vi "Test v2 Client.vi"() -> ()   [LabVIEW 2020]
uses:
  InfluxDB v2 Client/Client/Header-Body Data.ctl
  InfluxDB v2 Client/Client/Error Handler/HTTP Status.ctl
  InfluxDB v2 Client/Client/DataBase Data.ctl
  InfluxDB v2 Client/Data Point/Tag.ctl
  Field Values.ctl
  InfluxDB v2 Client/Client/Write Precision.ctl
  InfluxDB v2 Client/Client/Influx Command.ctl
  Setup/Setup Data.ctl
  InfluxDB v2 Client/Data Point/Data Point - Cmd.ctl
  InfluxDB v2 Client/Client/Write Data.ctl
  <vilib>/Utility/xml.llb/Read From XML File(string).vi
  <vilib>/Utility/xml.llb/Write to XML File(string).vi
  InfluxDB v2 Client/InfluxDB v2 Client.lvlib
panel:
  out "Response":T1
  in  "Tab Control":enum32{"Setup", "Init ", "Write", "Query"}(tab)
  in  "Write Setup":bool
  in  "Read Setup":bool
  in  "File Path Setup":path
  in  "Init":bool
  in  "Check Auth":bool
  in  "DataBase Data":T2
  in  "Timestamp precision":T3=enum."Seconds"
  in  "Measurement":string
  in  "Bucket":string
  in  "Init Data Point":bool
  in  "Write Data":bool
  in  "Field Names":string[](array[string])=["cpu_temp", "error_code", "cpu_load", "cpu_type", "cpu_busy"]
  in  "Tags":T4[](array[typedef])=[{"Key"="host1", "Value"="myPC"}, {"Key"="host2", "Value"="X-Server"}]
  in  "Field Values":T5={"cpu_temp"=48.25, "error_code"=-9003, "cpu_load"=8, "cpu_type"="Ryzen 5 2600", "cpu_busy?"=FALSE}
  in  "Write Query":bool
  in  "Read Query":bool
  in  "with compression?":bool
  in  "Write csv - file":bool
  in  "Query":string="from(bucket: \"Test\")\n  |> range(start: -30m)\n  |> filter(fn: (r) => r[\"_measurement\"] == \"mem3\")\n  |> filter(fn: (r) => r[\"_field\"] == \"cpu_temp\")\n  |> aggregateWindow(every: 1s, fn: last, createEmpty: false)\n  |> yield(name: \"last\")"
  in  "Query Data":bool
  in  "File Path Queries":path
  out "HTTP Status":T6
  in  "Stop":bool
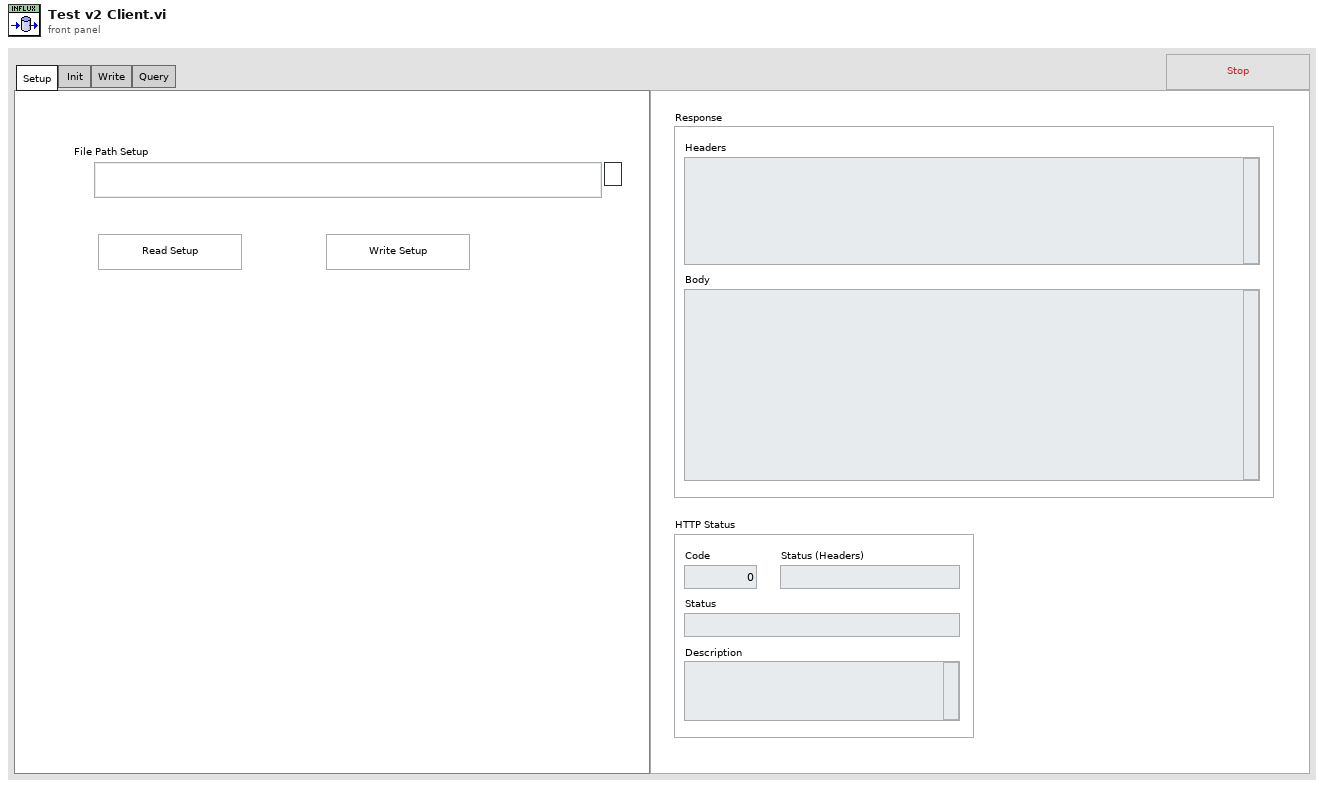
[diagram p1: front panel]
types:
  T1 = typedef "InfluxDB v2 Client.lvlib/Header-Body Data.ctl" = cluster{"Headers":string, "Body":string}
  T2 = typedef "InfluxDB v2 Client.lvlib/DataBase Data.ctl" = cluster{"Api Token":string, "Organization":string, "url":string, "Organization ID":string}
  T3 = typedef "InfluxDB v2 Client.lvlib/Write Precision.ctl" = enum16{"Nanoseconds", "Microseconds", "Milliseconds", "Seconds"}
  T4 = typedef "InfluxDB v2 Client.lvlib/Tag.ctl" = cluster{"Key":string, "Value":string}
  T5 = typedef "Field Values.ctl" = cluster{"cpu_temp":dbl, "error_code":i64, "cpu_load":u64, "cpu_type":string, "cpu_busy?":bool}
  T6 = typedef "InfluxDB v2 Client.lvlib/HTTP Status.ctl" = cluster{"Code":i32, "Status":string, "Description":string, "Status (Headers)":string}
  T7 = typedef "InfluxDB v2 Client.lvlib/Influx Command.ctl" = enum16{"Init", "Check Auth", "Query Data", "Query ZIP Data", "Write Data", "Close"}
  T8 = enum16{"open", "replace", "create", "open or create", "replace or create", "replace or create with confirmation"}
  T9 = typedef "InfluxDB v2 Client.lvlib/Data Point - Cmd.ctl" = enum16{"Init", "Add Tags", "Add Fields", "Add Field Names", "Add Field Values", "Add Measurement", "Add Time Stamp", "Add Precision", "Get Line Protocol"}
  T10 = typedef "Setup Data.ctl" = cluster{"DataBase Data":T2, "Query - csv":string, "Bucket":string, "Measurement":string, "Timestamp precision":T3, "Tags":T4[]}
  T11 = typedef "InfluxDB v2 Client.lvlib/Write Data.ctl" = cluster{"Bucket":string, "Timestamp precision":T3, "Line protocol":string}
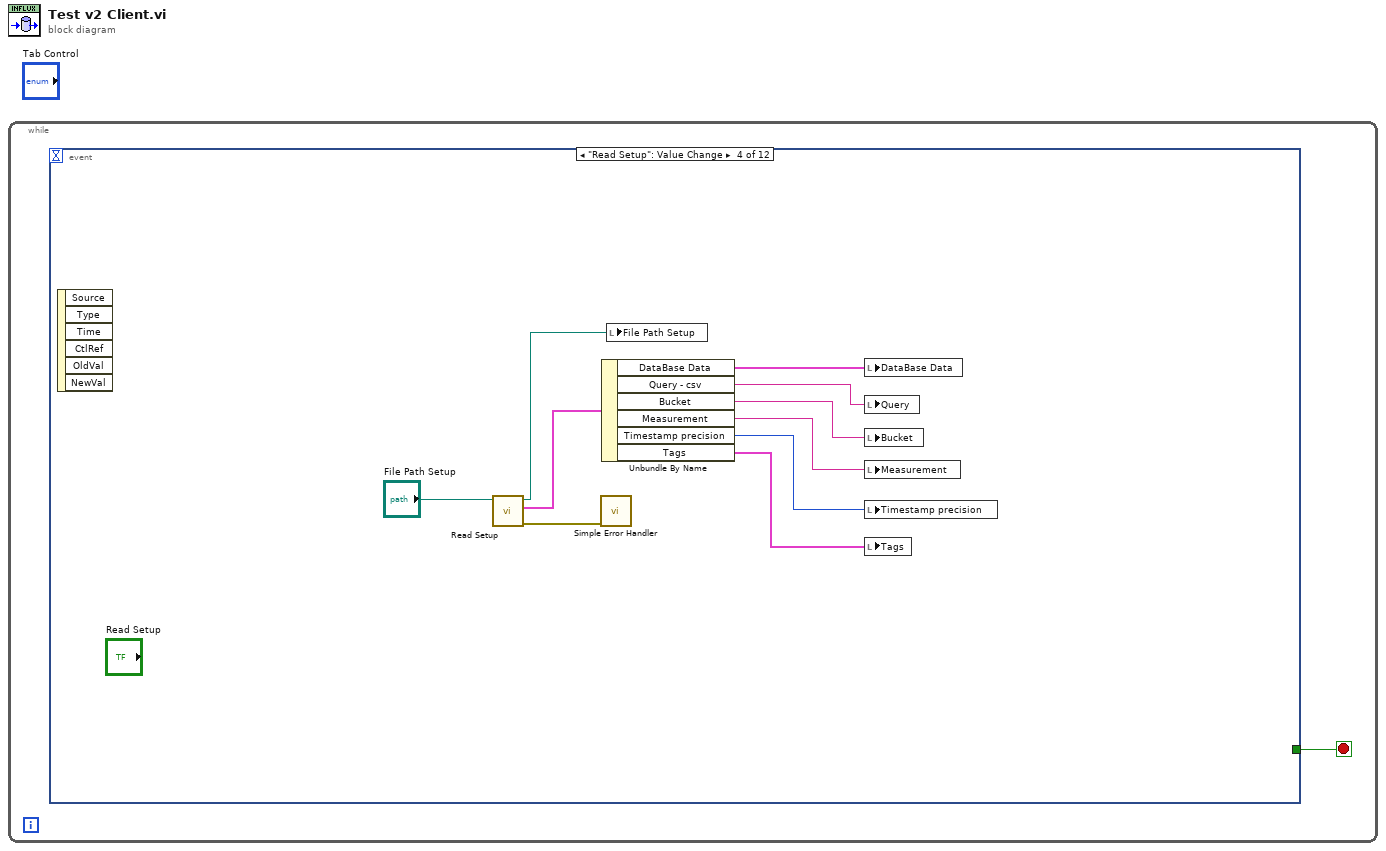
[diagram p0: block diagram]
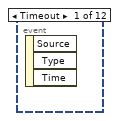
[diagram p2: hidden frame]
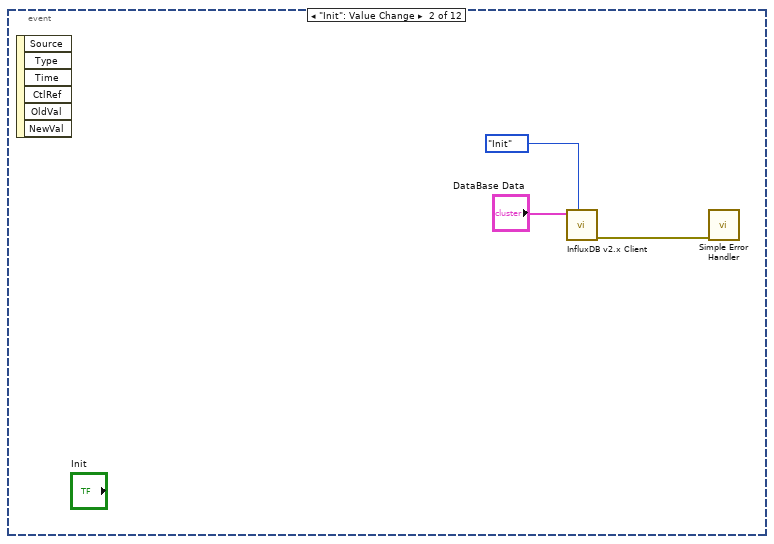
[diagram p3: hidden frame]
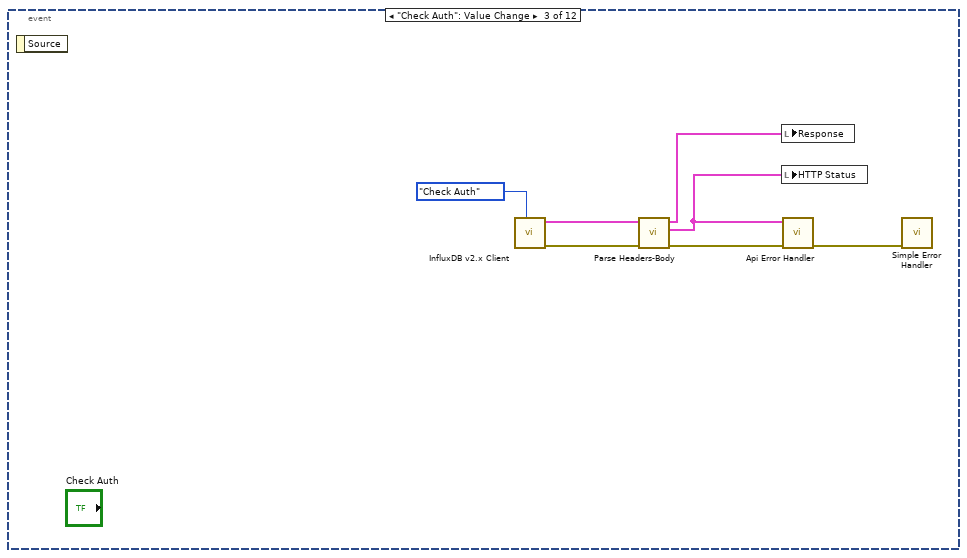
[diagram p4: hidden frame]
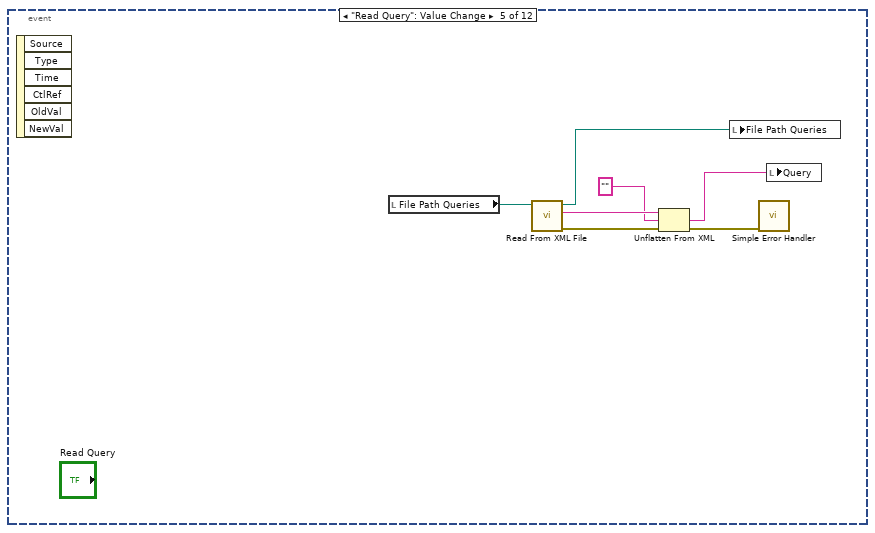
[diagram p5: hidden frame]
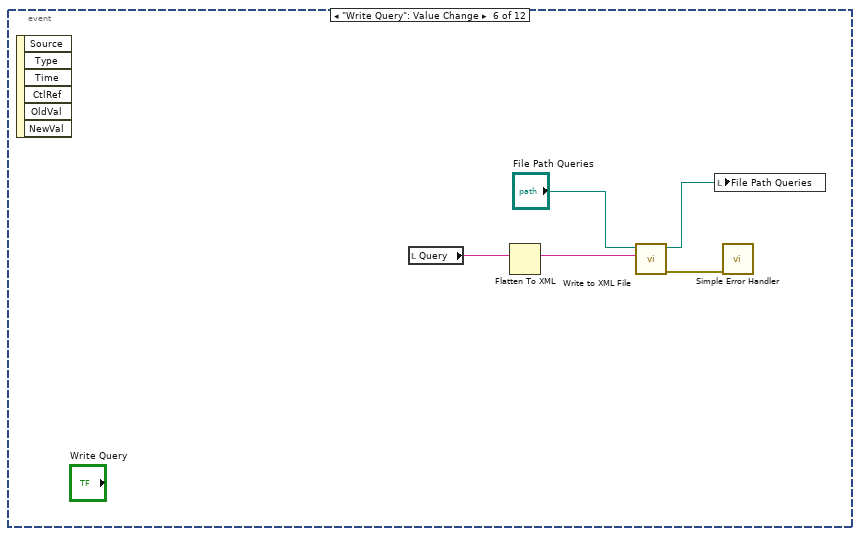
[diagram p6: hidden frame]
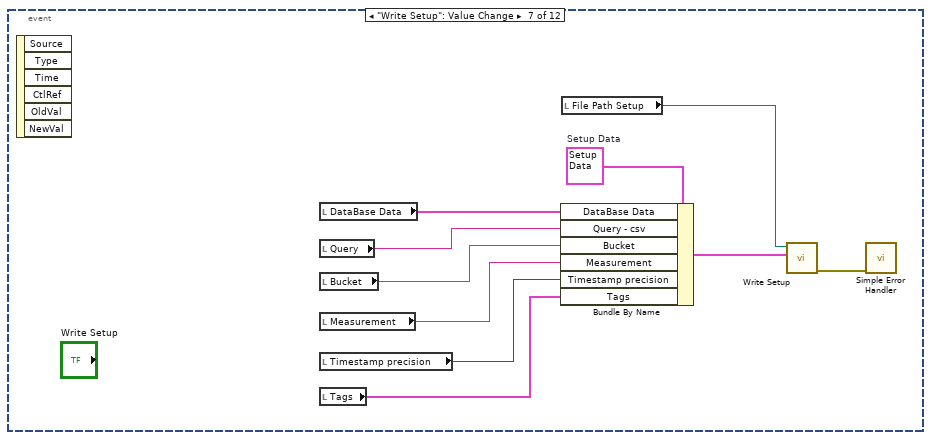
[diagram p7: hidden frame]
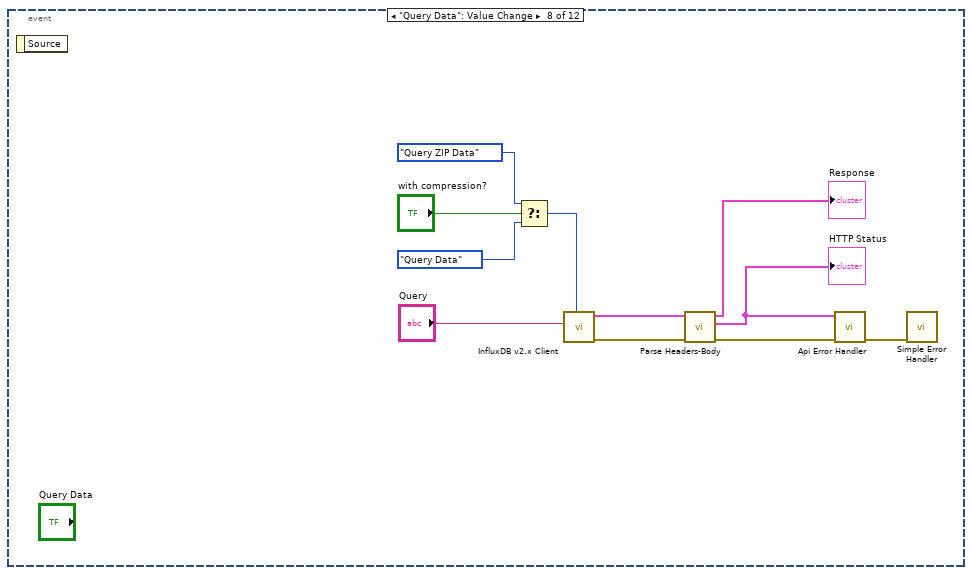
[diagram p8: hidden frame]
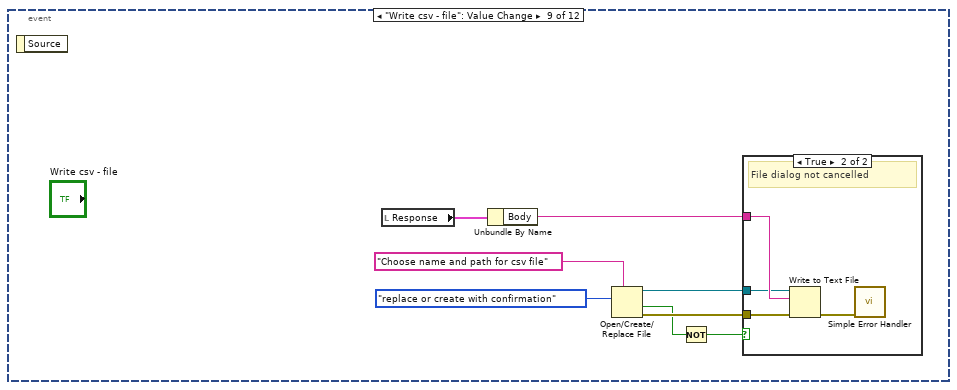
[diagram p9: hidden frame]
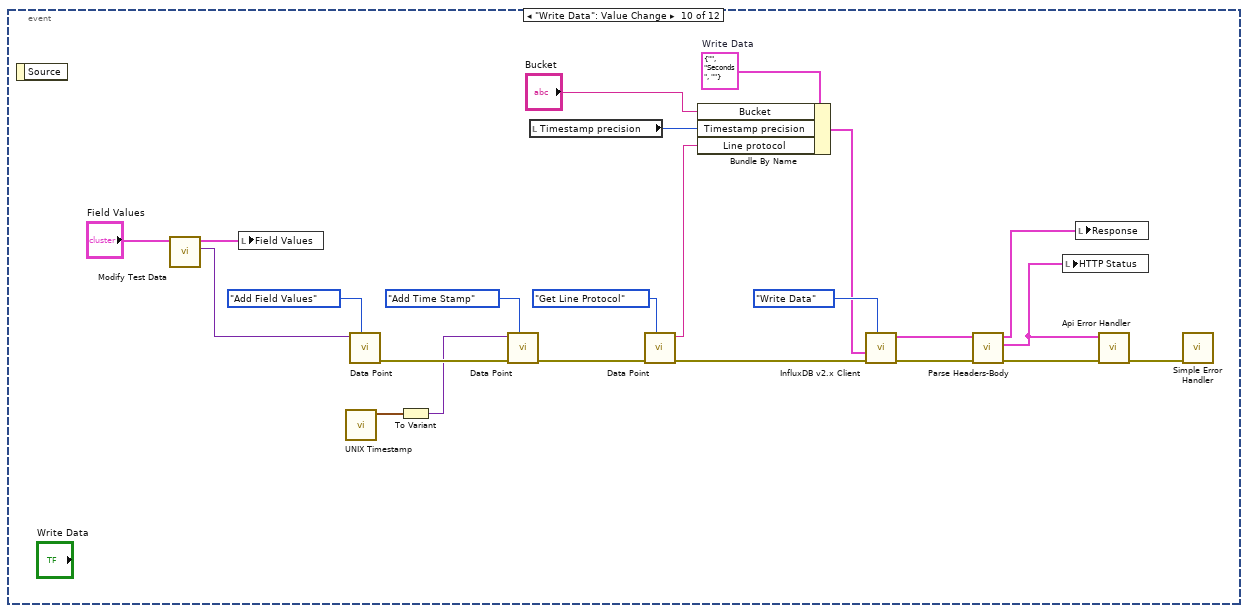
[diagram p11: hidden frame]
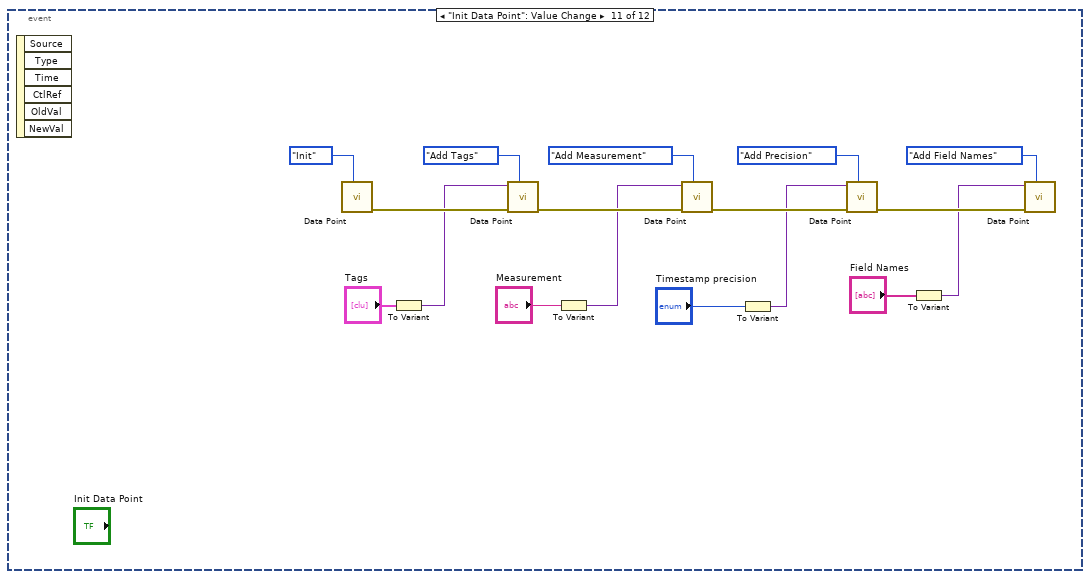
[diagram p12: hidden frame]
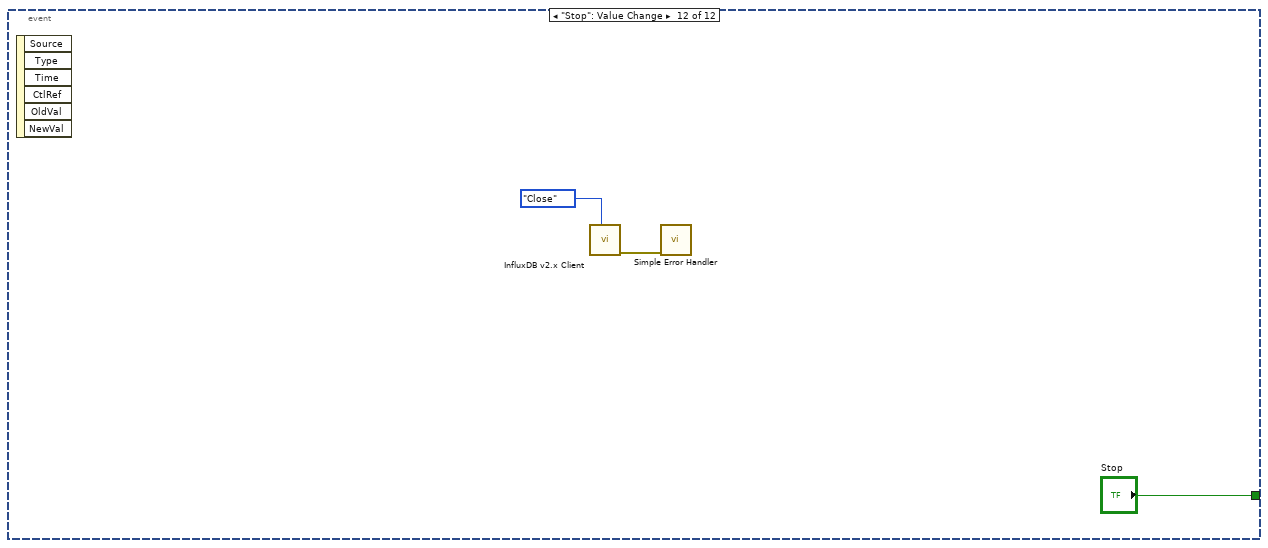
[diagram p13: hidden frame]
diagram:
  n1 = while {
    stop <- w1 stop-if-true
    n2 = event shown="[3] \"Read Setup\": Value Change" {
      selector: _ -> [_ _ _ _ _ _ _ _ _ _ _ _]
      dyn-events: _ -> [_ _ _ _ _ _ _ _ _ _ _ _]
      timeout: _ -> [_ _ _ _ _ _ _ _ _ _ _ _]
      tunnel: [_ _ _ _ _ _ _ _ _ _ _ "Stop"] -> w1
      event Timeout {
        n3 = event-data() -> ()  [unwired: 1 in, 3 out]
      }
      event "Init": Value Change {
        n4 = event-data() -> ()  [unwired: 1 in, 6 out]
        n5 = call "InfluxDB v2.x Client.vi"("Influx Command"=Influx_Command."Init", "DataBase Data"="DataBase Data") -> ("error out"=w3:errorcluster)  [unwired: 8 in, 1 out]
        n6 = call <vilib>:"Simple Error Handler.vi"("error in (no error)"=w3) -> ()  [unwired: 4 in, 5 out]
      }
      event "Check Auth": Value Change {
        n7 = event-data() -> ()  [unwired: 1 in, 1 out]
        n8 = call "InfluxDB v2.x Client.vi"("Influx Command"=Influx_Command."Check Auth") -> ("error out"=w9:errorcluster, "Header-Body Data"=w7:T1)  [unwired: 9 in]
        n9 = call "Parse Headers-Body.vi"("error in"=w9, "Header-Body Data in"=w7) -> ("error out"=w8:errorcluster, "HTTP Status"=w5:T6, "Header-Body Data out"=w6:T1)  [unwired: 7 in]
        n10 = local write "Response"(w6) -> ()
        n11 = local write "HTTP Status"(w5) -> ()
        n12 = call "Api Error Handler.vi"("error in"=w8, "HTTP Status"=w5) -> ("error out"=w10:errorcluster)  [unwired: 9 in]
        n13 = call <vilib>:"Simple Error Handler.vi"("error in (no error)"=w10) -> ()  [unwired: 4 in, 5 out]
      }
      event "Read Setup": Value Change {
        n14 = event-data() -> ()  [unwired: 1 in, 6 out]
        n15 = call "Read Setup.vi"("File Path in"="File Path Setup") -> ("error out"=w19:errorcluster, "Setup Data"=w13:T10, "File Path out"=w18:path)  [unwired: 8 in]
        n16 = call <vilib>:"Simple Error Handler.vi"("error in (no error)"=w19) -> ()  [unwired: 4 in, 5 out]
        n17 = Unbundle By Name(w13) -> ("DataBase Data"=w20:T2, "Query - csv"=w17:string, "Bucket"=w16:string, "Measurement"=w15:string, "Timestamp precision"=w14:T3, "Tags"=w12:T4[])
        n18 = local write "File Path Setup"(w18) -> ()
        n19 = local write "DataBase Data"(w20) -> ()
        n20 = local write "Query"(w17) -> ()
        n21 = local write "Bucket"(w16) -> ()
        n22 = local write "Measurement"(w15) -> ()
        n23 = local write "Timestamp precision"(w14) -> ()
        n24 = local write "Tags"(w12) -> ()
      }
      event "Read Query": Value Change {
        n25 = event-data() -> ()  [unwired: 1 in, 6 out]
        n26 = local read "File Path Queries"() -> (w28:path)
        n27 = call-poly <vilib>:"Read From XML File.vi"("XML File Path"=w28) -> ("error out"=w26:errorcluster, "XML Elements"=w25:string, "XML File Path(duplicate)"=w27:path)  [unwired: 8 in]
        n28 = Unflatten From XML(xml string=w25, type="", error in (no error)=w26) -> (value=w23:string, error out=w22:errorcluster)
        n29 = local write "File Path Queries"(w27) -> ()
        n30 = call <vilib>:"Simple Error Handler.vi"("error in (no error)"=w22) -> ()  [unwired: 4 in, 5 out]
        n31 = local write "Query"(w23) -> ()
      }
      event "Write Query": Value Change {
        n32 = event-data() -> ()  [unwired: 1 in, 6 out]
        n33 = local read "Query"() -> (w33:string)
        n34 = Flatten To XML(6:w33) -> (2:w32:string)
        n35 = call-poly <vilib>:"Write to XML File.vi"("XML Input"=w32, "XML File Path"="File Path Queries") -> ("error out"=w29:errorcluster, "XML File Path(duplicate)"=w30:path)  [unwired: 7 in, 1 out]
        n36 = local write "File Path Queries"(w30) -> ()
        n37 = call <vilib>:"Simple Error Handler.vi"("error in (no error)"=w29) -> ()  [unwired: 4 in, 5 out]
      }
      event "Write Setup": Value Change {
        w43 = T10 {"DataBase Data"={"Api Token"="", "Organization"="", "url"="", "Organization ID"=""}, "Query - csv"="", "Bucket"="", "Measurement"="", "Timestamp precision"=enum."Seconds", "Tags"=[{"Key"="host1", "Value"="myPC"}, {"Key"="host2", "Value"="X-Server"}]}  # Setup Data
        n38 = event-data() -> ()  [unwired: 1 in, 6 out]
        n39 = local read "DataBase Data"() -> (w42:T2)
        n40 = local read "Query"() -> (w38:string)
        n41 = local read "Bucket"() -> (w37:string)
        n42 = local read "Measurement"() -> (w36:string)
        n43 = local read "Timestamp precision"() -> (w35:T3)
        n44 = local read "Tags"() -> (w34:T4[])
        n45 = Bundle By Name(cluster=w43, "DataBase Data"=w42, "Query - csv"=w38, "Bucket"=w37, "Measurement"=w36, "Timestamp precision"=w35, "Tags"=w34) -> (w40:T10)
        n46 = local read "File Path Setup"() -> (w41:path)
        n47 = call "Write Setup.vi"("Setup Data"=w40, "File Path"=w41) -> ("error out"=w39:errorcluster)  [unwired: 9 in]
        n48 = call <vilib>:"Simple Error Handler.vi"("error in (no error)"=w39) -> ()  [unwired: 4 in, 5 out]
      }
      event "Query Data": Value Change {
        n49 = event-data() -> ()  [unwired: 1 in, 1 out]
        n50 = Select(t=Influx_Command."Query ZIP Data" ("Influx Command"), s="with compression?", f=Influx_Command."Query Data" ("Influx Command")) -> (s? t:f=w49:T7)
        n51 = call "InfluxDB v2.x Client.vi"("Influx Command"=w49, "Query Data"="Query") -> ("error out"=w48:errorcluster, "Header-Body Data"=w47:T1)  [unwired: 8 in]
        n52 = call "Parse Headers-Body.vi"("error in"=w48, "Header-Body Data in"=w47) -> ("error out"=w46:errorcluster, "HTTP Status"=w44:T6, "Header-Body Data out"=→"Response":T1)  [unwired: 7 in]
        "HTTP Status" <- w44
        n53 = call "Api Error Handler.vi"("error in"=w46, "HTTP Status"=w44) -> ("error out"=w54:errorcluster)  [unwired: 9 in]
        n54 = call <vilib>:"Simple Error Handler.vi"("error in (no error)"=w54) -> ()  [unwired: 4 in, 5 out]
      }
      event "Write csv - file": Value Change {
        n55 = event-data() -> ()  [unwired: 1 in, 1 out]
        n56 = local read "Response"() -> (w62:T1)
        n57 = Unbundle By Name(w62) -> ("Body"=w61:string)
        n58 = Open/Create/Replace File(prompt="Choose name and path for csv file" ("prompt (Choose or enter file path)"), operation (0:open)=T8."replace or create with confirmation") -> (refnum out=w57:refnum<file>, cancelled=w56:bool, error out=w58:errorcluster)  [unwired: 4 in]
        n59 = Not(x=w56) -> (.not. x?=w55:bool)
        n60 = case shown="True" w55 {
          tunnel: w61 -> [_ w66]
          tunnel: w58 -> [_ w65]
          tunnel: w57 -> [_ w64]
          frame False {
          }
          frame True {
            # "File dialog not cancelled"
            n61 = Write to Text File(file (use dialog)=w64, text=w66, error in=w65) -> (error out=w63:errorcluster)  [unwired: 1 in, 2 out]
            n62 = call <vilib>:"Simple Error Handler.vi"("error in (no error)"=w63) -> ()  [unwired: 4 in, 5 out]
          }
        }
      }
      event "Write Data": Value Change {
        w71 = T11 {"Bucket"="", "Timestamp precision"=enum."Seconds", "Line protocol"=""}  # Write Data
        n63 = event-data() -> ()  [unwired: 1 in, 1 out]
        n64 = call "Modify Test Data.vi"("Field Values in"="Field Values") -> ("Variant"=w77:variant, "Field Values out"=w78:T5)  [unwired: 9 in]
        n65 = local write "Field Values"(w78) -> ()
        n66 = call "UNIX Timestamp.vi"() -> ("UNIX Time Stamp"=w81:timestamp)  [unwired: 11 in]
        n67 = call "Data Point.vi"("Data Point - Cmd"=Data_Point_-_Cmd."Add Field Values", "Data"=w77) -> ("error out"=w85:errorcluster)  [unwired: 8 in, 1 out]
        n68 = To Variant(anything=w81) -> (Variant=w82:variant)
        n69 = call "Data Point.vi"("Data Point - Cmd"=Data_Point_-_Cmd."Add Time Stamp", "error in"=w85, "Data"=w82) -> ("error out"=w83:errorcluster)  [unwired: 7 in, 1 out]
        n70 = local read "Timestamp precision"() -> (w69:T3)
        n71 = call "Data Point.vi"("Data Point - Cmd"=Data_Point_-_Cmd."Get Line Protocol", "error in"=w83) -> ("error out"=w80:errorcluster, "Line protocol"=w68:string)  [unwired: 8 in]
        n72 = Bundle By Name(cluster=w71, "Bucket"="Bucket", "Timestamp precision"=w69, "Line protocol"=w68) -> (w67:T11)
        n73 = call "InfluxDB v2.x Client.vi"("Influx Command"=Influx_Command."Write Data", "error in"=w80, "Write Data"=w67) -> ("error out"=w76:errorcluster, "Header-Body Data"=w74:T1)  [unwired: 7 in]
        n74 = call "Parse Headers-Body.vi"("error in"=w76, "Header-Body Data in"=w74) -> ("error out"=w75:errorcluster, "HTTP Status"=w72:T6, "Header-Body Data out"=w73:T1)  [unwired: 7 in]
        n75 = local write "HTTP Status"(w72) -> ()
        n76 = local write "Response"(w73) -> ()
        n77 = call "Api Error Handler.vi"("error in"=w75, "HTTP Status"=w72) -> ("error out"=w88:errorcluster)  [unwired: 9 in]
        n78 = call <vilib>:"Simple Error Handler.vi"("error in (no error)"=w88) -> ()  [unwired: 4 in, 5 out]
      }
      event "Init Data Point": Value Change {
        n79 = event-data() -> ()  [unwired: 1 in, 6 out]
        n80 = call "Data Point.vi"("Data Point - Cmd"=Data_Point_-_Cmd."Init") -> ("error out"=w105:errorcluster)  [unwired: 9 in, 1 out]
        n81 = To Variant(anything="Tags") -> (Variant=w102:variant)
        n82 = call "Data Point.vi"("Data Point - Cmd"=Data_Point_-_Cmd."Add Tags", "error in"=w105, "Data"=w102) -> ("error out"=w101:errorcluster)  [unwired: 7 in, 1 out]
        n83 = To Variant(anything="Measurement") -> (Variant=w99:variant)
        n84 = call "Data Point.vi"("Data Point - Cmd"=Data_Point_-_Cmd."Add Measurement", "error in"=w101, "Data"=w99) -> ("error out"=w98:errorcluster)  [unwired: 7 in, 1 out]
        n85 = To Variant(anything="Timestamp precision") -> (Variant=w96:variant)
        n86 = call "Data Point.vi"("Data Point - Cmd"=Data_Point_-_Cmd."Add Precision", "error in"=w98, "Data"=w96) -> ("error out"=w95:errorcluster)  [unwired: 7 in, 1 out]
        n87 = To Variant(anything="Field Names") -> (Variant=w92:variant)
        n88 = call "Data Point.vi"("Data Point - Cmd"=Data_Point_-_Cmd."Add Field Names", "error in"=w95, "Data"=w92) -> ()  [unwired: 7 in, 2 out]
      }
      event "Stop": Value Change {
        n89 = event-data() -> ()  [unwired: 1 in, 6 out]
        n90 = call "InfluxDB v2.x Client.vi"("Influx Command"=Influx_Command."Close") -> ("error out"=w107:errorcluster)  [unwired: 9 in, 1 out]
        n91 = call <vilib>:"Simple Error Handler.vi"("error in (no error)"=w107) -> ()  [unwired: 4 in, 5 out]
      }
    }
  }
